vi "Get Actor List.vi"(8 "error in (no error)":errorcluster, 11 "Actor Store":refnum<class "Actor Store.lvclass">) -> (0 "Actor Label":string, 1 "Actors":string[](array[string]), 2 "Actor Paths":variant, 3 "Actor Store":refnum<class "Actor Store.lvclass">)   [LabVIEW 2023, in "Add Async Methods Actor.lvlib"]
uses:
  Add Async Methods Actor.lvlib
  Classes/Actor Store/Actor Store.lvclass
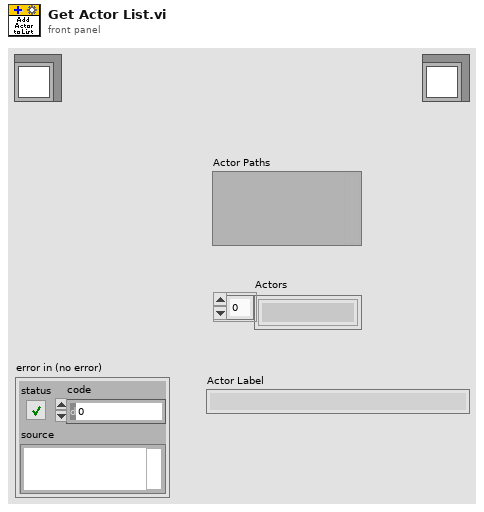
[diagram p1: front panel]
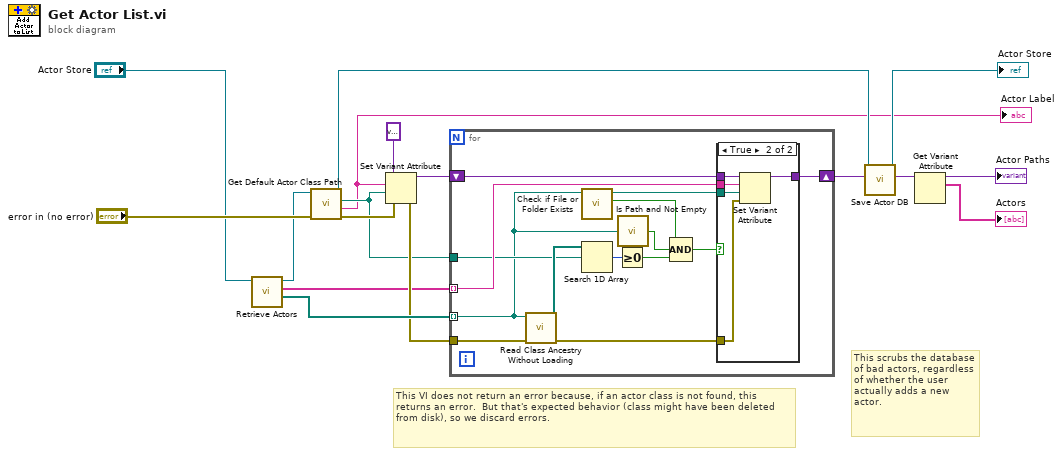
[diagram p0: block diagram]
diagram:
  # "This scrubs the database of bad actors, regardless of whether the user actually adds a new actor."
  # "This VI does not return an error because, if an actor class is not found, this returns an error.  But that's expected behavior (class might have been deleted from disk), so we discard errors."
  n1 = call-dynamic "Retrieve Actors.vi"("Actor Store in"="Actor Store") -> ("Actor Paths"=w15:path[], "Actors"=w2:string[], "Actor Store out"=w8:refnum<class "Actor Store.lvclass">)  [unwired: 7 in, 1 out]
  n2 = call "Get Default Actor Class Path.vi"("error in (no error)"="error in (no error)", "Actor Store"=w8) -> ("error out"=w14:errorcluster, "Actor Label"=w1:string, "Path String"=w9:path, "Actor Store"=w4:refnum<class "Actor Store.lvclass">)  [unwired: 6 in]
  "Actor Label" <- w1
  n3 = Set Variant Attribute(Variant=variant ("variant"), name=w1, value=w9, error in=w14) -> (Variant out=w17:variant, error out=w13:errorcluster)  [unwired: 1 out]
  n4 = for {
    tunnel: w2 -> [w29] mode=indexing
    shift-right: [w31] -> w6
    shift-left: w17 -> [w30]
    tunnel: w15 -> [w19] mode=indexing
    tunnel: w9 -> [w24]
    tunnel: w13 -> [w26]
    n5 = call <vilib>:"Read Class Ancestry Without Loading.vi"("error in (no error)"=w26, "LabVIEW Class Path"=w19) -> ("error out"=w25:errorcluster, "Class Ancestry"=w28:path[])  [unwired: 8 in]
    n6 = call <vilib>:"Check if File or Folder Exists.vi"("path"=w19) -> ("file or folder exists?"=w21:bool, "dup path"=w20:path)  [unwired: 8 in, 1 out]
    n7 = Search 1D Array(1D array=w28, element=w24) -> (index of element=w27:i32)  [unwired: 1 in]
    n8 = Greater Or Equal To 0?(x=w27) -> (x >= 0?=w23:bool)
    n9 = call <vilib>:"Is Path and Not Empty.vi"("path"=w19) -> ("Is Path and Not Empty?"=w18:bool)  [unwired: 4 in]
    n10 = Compound Arithmetic op=AND(w21, w18, w23) -> (w22:bool)
    n11 = case shown="True" w22 {
      tunnel: [w32 w37] -> w31
      tunnel: w30 -> [w32 w36]
      tunnel: w29 -> [_ w35]
      tunnel: w25 -> [_ w34]
      tunnel: w20 -> [_ w33]
      frame False {
      }
      frame True {
        n12 = Set Variant Attribute(Variant=w36, name=w35, value=w33, error in=w34) -> (Variant out=w37:variant)  [unwired: 2 out]
      }
    }
  }
  n13 = call "Save Actor DB.vi"("Actor DB"=w6, "Actor Store"=w4) -> ("Actor DB Out"=w5:variant, "Actor Store"=→"Actor Store":refnum<class "Actor Store.lvclass">)  [unwired: 7 in, 1 out]
  n14 = Get Variant Attribute(Variant=w5) -> (duplicate Variant=→"Actor Paths":variant, names=→"Actors":string[])  [unwired: 3 in, 2 out]
